vi "uService GUI.vi"(8 "error in (no error)":errorcluster, 11 "uService Template in":refnum<class "New uService Template.lvclass">) -> (3 "uService Template out":refnum<class "New uService Template.lvclass">)   [LabVIEW 2021, in "New uService Template.lvlib" / "New uService Template.lvclass"]
uses:
  New uService Template.lvclass
  TALOS/TALOS_PPL.lvlibp/Father of all uServices/Father of all uServices/Father of all uServices.lvclass
  C:/LabVIEW Code/aegis-labview-code/TALOS/TALOS_PPL.lvlibp/Father of all uServices/Father of all uServices/Father of all uServices.lvclass
panel:
  in  "stop New uService":bool
  in  "Example":bool
  # "I'm the new uService!"
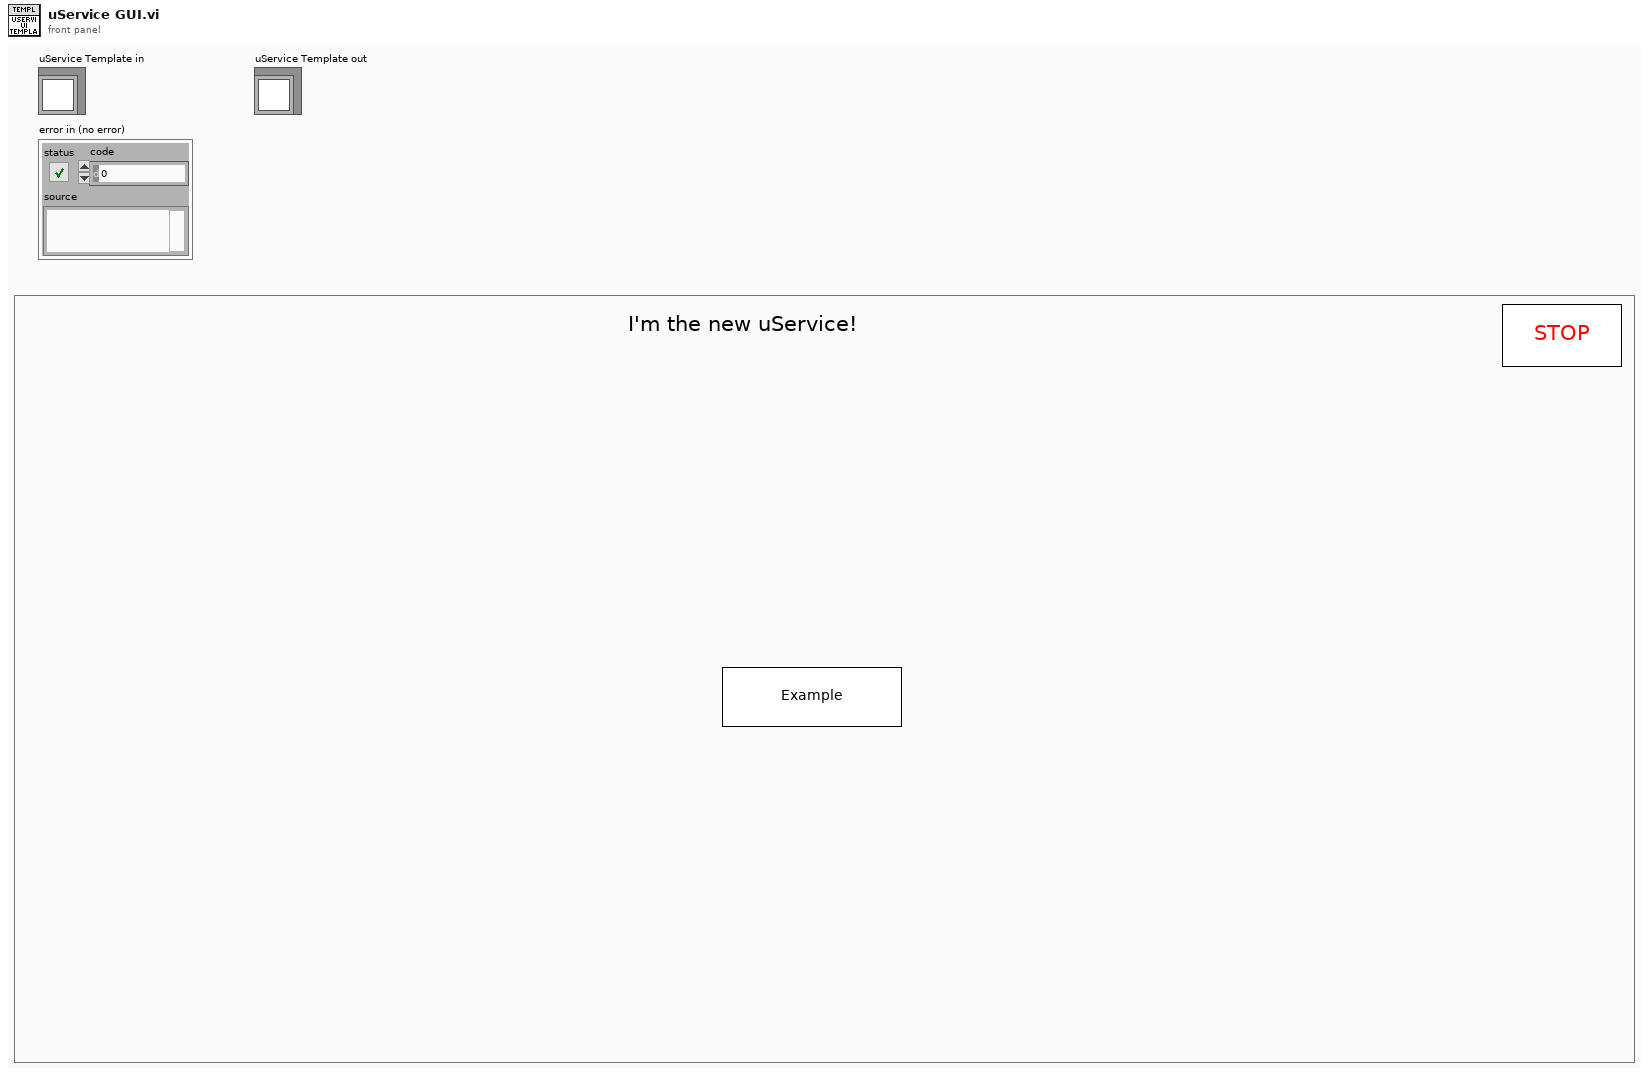
[diagram p1: front panel]
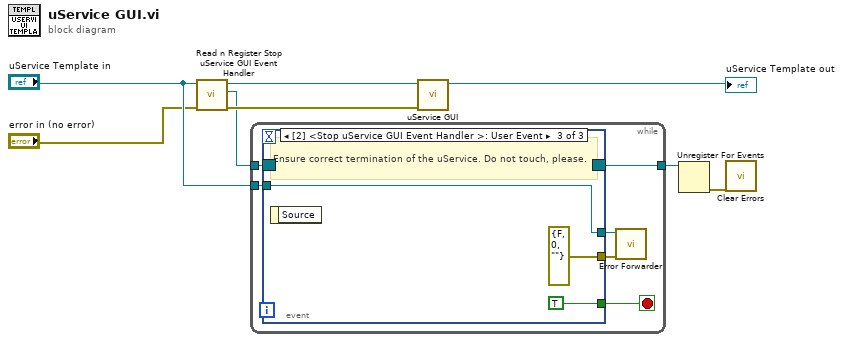
[diagram p0: block diagram]
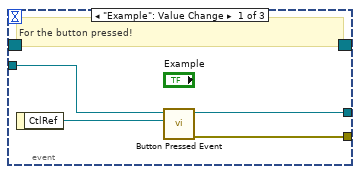
[diagram p2: hidden frame]
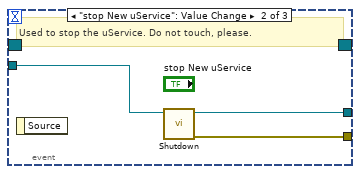
[diagram p3: hidden frame]
diagram:
  n1 = call-dynamic "Read n Register Stop uService GUI Event Handler .vi"("error in (no error)"="error in (no error)", "uService Template in"="uService Template in") -> ("error out"=w6:errorcluster, "Stop uService GUI Event Ref"=w5:refnum<event-registration>, "uService Template out"=w7:refnum<class "New uService Template.lvclass">)  [unwired: 7 in]
  n2 = while {
    tunnel: [w14] -> w8
    tunnel: w5 -> [w12]
    tunnel: "uService Template in" -> [w11]
    stop <- w13 stop-if-true
    n3 = event shown="[2] <Stop uService GUI Event Handler >: User Event" {
      selector: w12 -> [_ _ _]
      dyn-events: [_ _ _] -> w14
      timeout: _ -> [_ _ _]
      tunnel: [_ _ TRUE] -> w13
      tunnel: w11 -> [w18 w21 w23]
      tunnel: [w16 w20 errorcluster {"status"=FALSE, "code"=0, "source"=""} ("error out")] -> w10
      tunnel: [w15 w19 w23] -> w9
      event "Example": Value Change {
        # "For the button pressed!"
        n4 = event-data() -> ("CtlRef"=w17:refnum<vi>)  [unwired: 1 in]
        n5 = call-dynamic "Button Pressed Event.vi"("CtlRef"=w17, "uService Template in"=w18) -> ("error out"=w16:errorcluster, "uService Template out"=w15:refnum<class "New uService Template.lvclass">)  [unwired: 8 in]
      }
      event "stop New uService": Value Change {
        # "Used to stop the uService. Do not touch, please."
        n6 = event-data() -> ()  [unwired: 1 in, 1 out]
        n7 = call "Shutdown.vi"("Father of all uServices in"=w21) -> ("error out"=w20:errorcluster, "Father of all uServices out"=w19:refnum<class "New uService Template.lvclass">)  [unwired: 9 in]
      }
      event User Event {
        # "Ensure correct termination of the uService. Do not touch, please."
        n8 = event-data() -> ()  [unwired: 1 in, 1 out]
      }
    }
    n9 = call "Error Forwarder.vi"("error in (no error)"=w10, "Father of all uServices in"=w9) -> ()  [unwired: 10 in]
  }
  n10 = call-parent "uService GUI.vi"("error in (no error)"=w6, "uService Template in"=w7) -> ("uService Template out"=→"uService Template out":refnum<class "New uService Template.lvclass">)  [unwired: 9 in]
  n11 = Unregister For Events(event registration refnum=w8) -> (error out=w1:errorcluster)  [unwired: 1 in]
  n12 = call <vilib>:"Clear Errors.vi"("error in (no error)"=w1) -> ()  [unwired: 5 in, 2 out]
